vi "find_goal_pose.vi"(6 "Reset":bool, 7 "Parameters":T2={"Stimulus"={"Type"=enum."Off", "Phase"=0.0, "Amplitude"=[], "Injection point"=enum."Total pose", "Closed loop"=FALSE, "Offset"=[], "Tip -> world"=FALSE, "Frequency"=0.0, "Length"=0.0}, "Goal Filter A"={"Speedup max"=0.0, "Speedup thresh"=0.0, "Speedup nonlin"=0.0, "Filters"=[]}, "Mode controls"={"Hold"=FALSE, "Cancellation"=FALSE, "Goal filter"=FALSE, "Trigger"=FALSE}, "Manipulator type"=enum."Current piezo", "Manipulator calibration"={"Tool offsets"=[[0.0, 0.0, 36200.0]], "Handle light calibration"=[], "Base pivots"=[], "Output pivots"=[], "Length center"=0.0, "Workspace height"=[], "Workspace diameter"=[0.0, 0.0, 36200.0], "Stack travel"=400.0, "Saturation pos"=375.0, "Inverse filters"=[], "Strut length"=0.0}, "Network"={"Remote Host"="", "Send Status"=FALSE, "Send Port"=0, "Recv Commands"=FALSE, "Recv Port"=0}, "Goal Filter B"={"Speedup max"=0.0, "Speedup thresh"=0.0, "Speedup nonlin"=0.0, "Filters"=[]}, "Cancellation"={"KP"={"XY"=0.0, "Rxy"=0.0, "Z"=0.0, "Rz"=0.0}, "KI"=0.0, "KD"={"XY"=0.0, "Rxy"=0.0, "Z"=0.0, "Rz"=0.0}, "Max vel"=20.0, "Max acc"=0.001, "Int error limit"=3.0, "RCM gain"=0.0, "Bypass"=FALSE, "Degraded gain"=0.0}, "Transition time"=0.0, "Estimation"={"Link"={"Measure noise"=[], "Process noise"=[], "Alt process noise"=[], "Alt turnoff cycles"=20, "Innovation limit"=[], "Residue threshold"=0.0, "Enable"=FALSE}, "Handle"={"Measure noise"=[], "Process noise"=[], "State limits"=[], "Innovation limit"=[], "Prediction Lookahead"=0.0, "Enable"=FALSE}}} {"Transition time" format="%_3f"; "Cancellation"."Degraded gain" min=0 max=1 step=0.1 format="%#_3p"; "Cancellation"."RCM gain" min=0 max=1 step=0.1 format="%#_3p"; "Cancellation"."KD"."Rz" min=-1 max=1 step=0.01 format="%#_3p"; "Cancellation"."KD"."Rxy" min=-1 max=1 step=0.01 format="%#_3p"; "Cancellation"."KD"."Z" min=-1 max=1 step=0.01 format="%#_3p"; "Cancellation"."KD"."XY" min=-1 max=1 step=0.01 format="%#_3p"; "Cancellation"."KI" min=0 max=1 step=0.01 format="%#_3p"; "Cancellation"."KP"."Rz" min=-1 max=1 step=0.01 format="%#_3p"; "Cancellation"."KP"."Rxy" min=-1 max=1 step=0.01 format="%#_3p"; "Cancellation"."KP"."Z" min=-1 max=1 step=0.01 format="%#_3p"; "Cancellation"."KP"."XY" min=-1 max=1 step=0.01 format="%#_3p"; "Cancellation"."Max acc" format="%#_3p"; "Goal Filter B"."Filters"."V limit range" format="%_3p"; "Goal Filter B"."Filters"."V limit" format="%_3p"; "Goal Filter B"."Filters"."Upper Q" format="%_3f"; "Goal Filter B"."Filters"."Upper Fc" format="%_3p"; "Goal Filter B"."Filters"."Lower Q" format="%_3f"; "Goal Filter B"."Filters"."Scale factor" format="%_3f"; "Goal Filter B"."Filters"."Lower Fc" format="%_3p"; "Goal Filter B"."Speedup nonlin" format="%_3p"; "Goal Filter B"."Speedup thresh" format="%_3p"; "Goal Filter B"."Speedup max" format="%_3p"; "Manipulator calibration"."Strut length" format="%#_4p"; "Manipulator calibration"."Saturation pos" format="%#.1f"; "Manipulator calibration"."Stack travel" format="%#.1f"; "Manipulator calibration"."Length center" format="%#_4p"; "Manipulator calibration"."Output pivots" format="%#_6f"; "Manipulator calibration"."Base pivots" format="%#_6f"; "Manipulator calibration"."Handle light calibration" format="%#.1f"; "Goal Filter A"."Filters"."V limit range" format="%_3p"; "Goal Filter A"."Filters"."V limit" format="%_3p"; "Goal Filter A"."Filters"."Upper Q" format="%_3f"; "Goal Filter A"."Filters"."Upper Fc" format="%_3p"; "Goal Filter A"."Filters"."Lower Q" format="%_3f"; "Goal Filter A"."Filters"."Scale factor" format="%_3f"; "Goal Filter A"."Filters"."Lower Fc" format="%_3p"; "Goal Filter A"."Speedup nonlin" format="%_3p"; "Goal Filter A"."Speedup thresh" format="%_3p"; "Goal Filter A"."Speedup max" format="%_3p"; "Stimulus"."Length" min=0.0 max=100.0 step=100.0 format="%#_4p"; "Stimulus"."Frequency" min=0.0 step=100.0 format="%#_4g"; "Stimulus"."Offset" format="%#_3p"; "Stimulus"."Amplitude" format="%#_3p"; "Stimulus"."Phase" min=-180.0 max=360.0 step=100.0 format="%#.2f"}, 10 "Goal position":sgl[][](array[numeric]) format="%#_6p") -> (0 "Saturation":bool[](array[boolean]), 2 "Goal pose":T1 format="%#_5g")   [LabVIEW 2014]
uses:
  testing/Micron params.ctl
  testing/stimulus.ctl
  testing/injection_point.ctl
  goal_loop_parms.ctl
  testing/mode_conrols.ctl
  testing/manipulator_cal.ctl
  asap/labview/testing/probe_calibration.ctl
  host/network_params.ctl
  cancellation/sq_control_params.ctl
  cancellation/decoupled_gain.ctl
  cancellation/estimation_controls.ctl
  <vilib>/Analysis/Matrix/Datatypes/RealMatrix.ctl
  <vilib>/Analysis/baseanly.llb/A x Vector.vi
  <vilib>/Analysis/baseanly.llb/Real A x B.vi
  <vilib>/Analysis/Matrix/Numeric/Conversions/Array To Matrix - RA2.vi
  <vilib>/Analysis/NI_AALBase.lvlib
  <vilib>/Analysis/Matrix/NI_Matrix.lvlib
panel:
  out "KC sat 2":bool[](array[boolean])
  out "Circle sat":bool
  out "KC sat 1":bool[](array[boolean])
  # "True if tip or RCM goal was moved to fit inside the workspace"
  # "Debug:"
  # "Find goal pose given tip and RCM goal points.   This is the output pose that we want the manipulator to move into.\nSee block diagram for details on how 6DOF pose is computed from this 5DOF information (given that the distance from RCM to tip is fixed.)  We also prevent manipulator saturation by compromising the goal to fit inside the design workspace.  This is distinct from the link-length goal substituion done by the position servo loop (which should be in effect for a most a short time if this code is working properly.)"
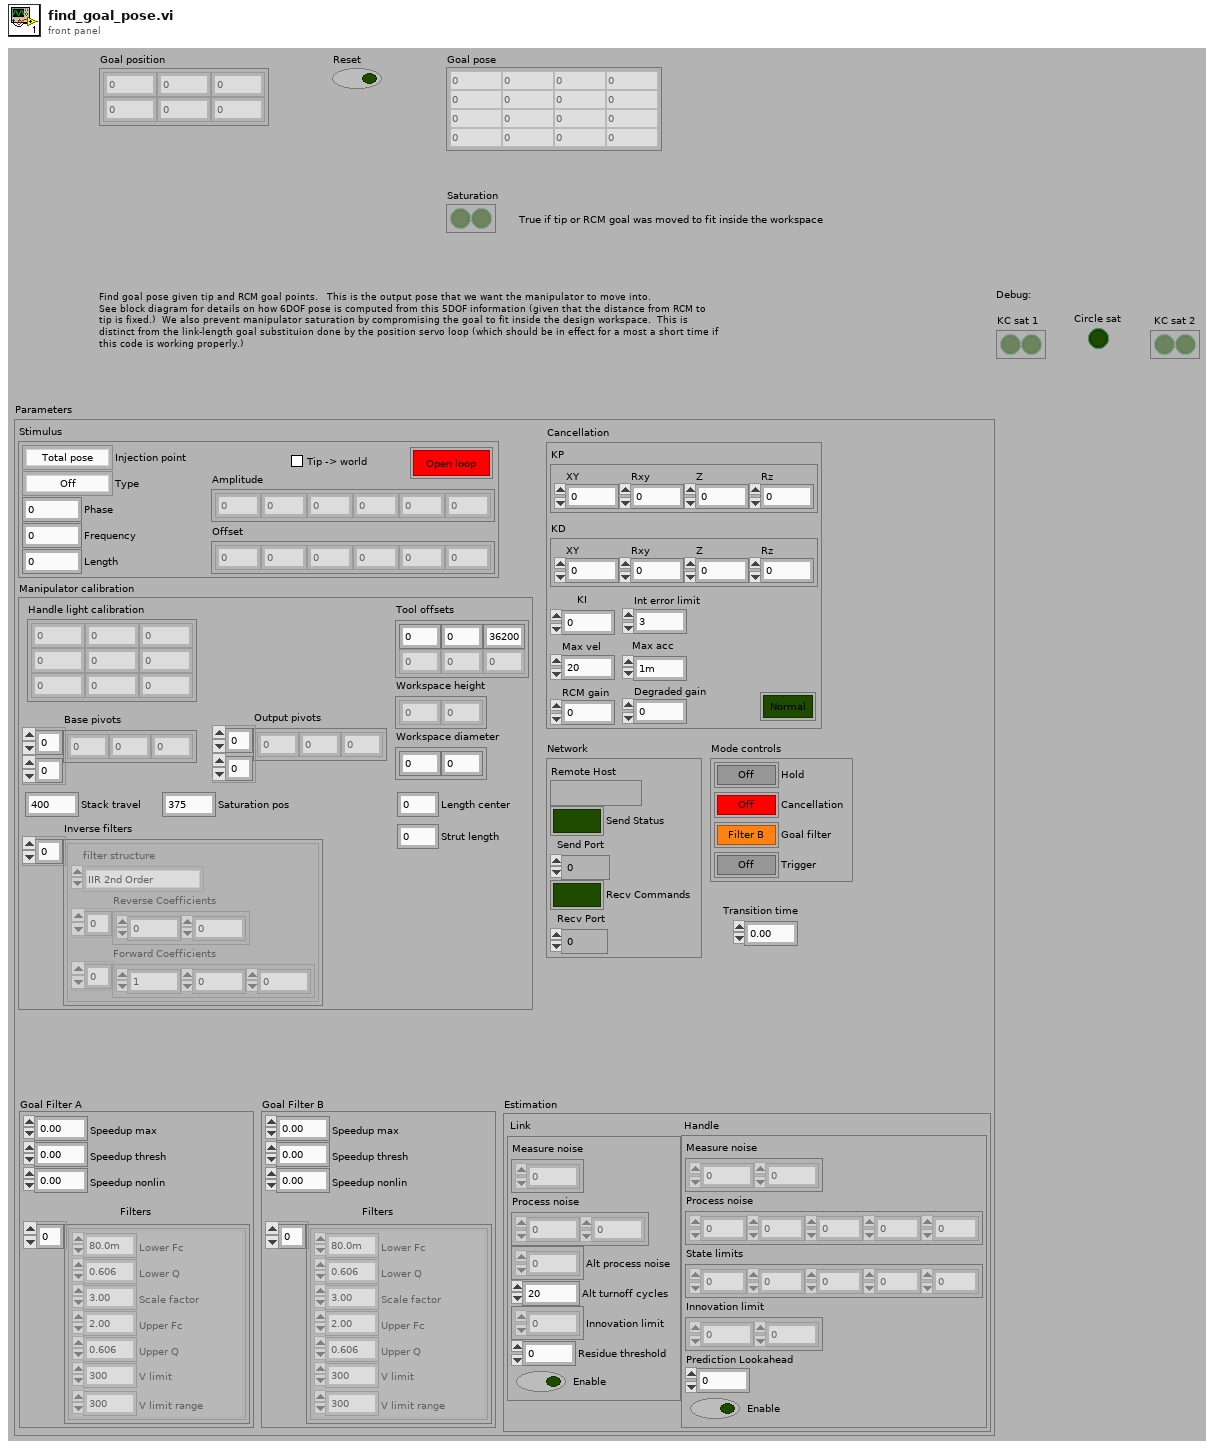
[diagram p1: front panel]
types:
  T1 = typedef "NI_Matrix.lvlib/RealMatrix.ctl" = dbl[][]
  T2 = typedef "Micron params.ctl" = cluster{"Stimulus":T3, "Goal Filter A":T5, "Mode controls":T6, "Manipulator type":enum16{"Current piezo", "Voltage piezo"}, "Manipulator calibration":T7, "Network":T9, "Goal Filter B":T5, "Cancellation":T10, "Transition time":sgl, "Estimation":T12}
  T3 = typedef "stimulus.ctl" = cluster{"Type":enum16{"Off", "Step", "Sine", "Triangle", "Arbitrary"}, "Phase":dbl, "Amplitude":sgl[], "Injection point":T4, "Closed loop":bool, "Offset":sgl[], "Tip -> world":bool, "Frequency":dbl, "Length":dbl}
  T4 = typedef "injection_point.ctl" = enum16{"Total pose", "V limiter", "Goal ", "Link position", "KF link position", "Inverse kin", "Link goal", "Link error", "Controller", "Output", "Drive", "Light"}
  T5 = typedef "goal_loop_parms.ctl" = cluster{"Speedup max":sgl, "Speedup thresh":sgl, "Speedup nonlin":sgl, "Filters":cluster{"Lower Fc":sgl, "Lower Q":sgl, "Scale factor":sgl, "Upper Fc":sgl, "Upper Q":sgl, "V limit":sgl, "V limit range":sgl}[]}
  T6 = typedef "mode_conrols.ctl" = cluster{"Hold":bool, "Cancellation":bool, "Goal filter":bool, "Trigger":bool}
  T7 = typedef "manipulator_cal.ctl" = cluster{"Tool offsets":sgl[][], "Handle light calibration":T8, "Base pivots":sgl[][], "Output pivots":sgl[][], "Length center":sgl, "Workspace height":sgl[], "Workspace diameter":sgl[], "Stack travel":sgl, "Saturation pos":sgl, "Inverse filters":cluster{"filter structure":enum32{"IIR 2nd Order", "IIR 4th Order"}, "Reverse Coefficients":dbl[], "Forward Coefficients":dbl[]}[], "Strut length":sgl}
  T8 = typedef "probe_calibration.ctl" = sgl[][]
  T9 = typedef "network_params.ctl" = cluster{"Remote Host":string, "Send Status":bool, "Send Port":u16, "Recv Commands":bool, "Recv Port":u16}
  T10 = typedef "sq_control_params.ctl" = cluster{"KP":T11, "KI":sgl, "KD":T11, "Max vel":sgl, "Max acc":sgl, "Int error limit":sgl, "RCM gain":sgl, "Bypass":bool, "Degraded gain":sgl}
  T11 = typedef "decoupled_gain.ctl" = cluster{"XY":sgl, "Rxy":sgl, "Z":sgl, "Rz":sgl}
  T12 = typedef "estimation_controls.ctl" = cluster{"Link":cluster{"Measure noise":dbl[], "Process noise":dbl[], "Alt process noise":dbl[], "Alt turnoff cycles":i32, "Innovation limit":dbl[], "Residue threshold":dbl, "Enable":bool}, "Handle":cluster{"Measure noise":dbl[], "Process noise":dbl[], "State limits":dbl[], "Innovation limit":dbl[], "Prediction Lookahead":sgl, "Enable":bool}}
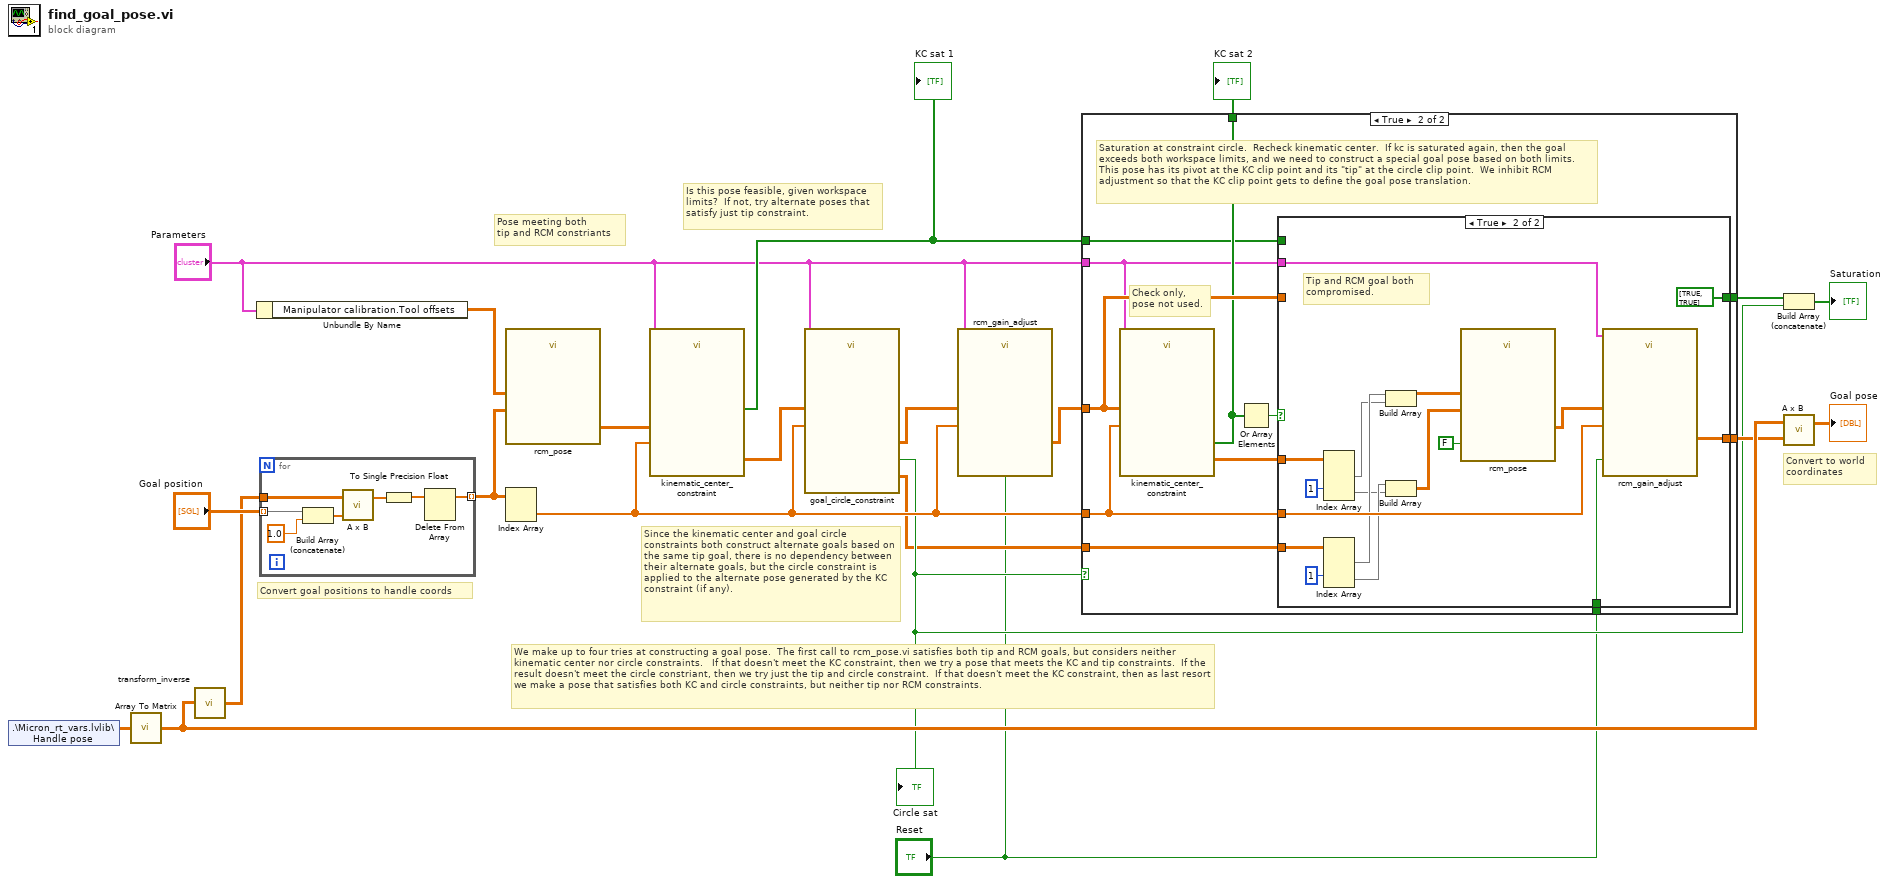
[diagram p0: block diagram]
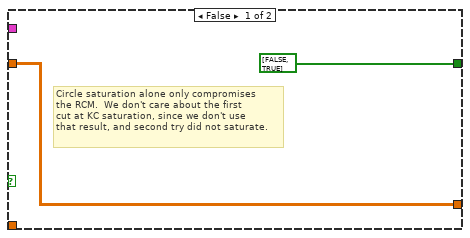
[diagram p3: hidden frame]
diagram:
  # "We make up to four tries at constructing a goal pose.  The first call to rcm_pose.vi satisfies both tip and RCM goals, but considers neither kinematic center nor circle constraints.   If that doesn't meet the KC constraint, then we try a pose that meets the KC and tip constraints.  If the result doesn't meet the circle constriant, then we try just the tip and circle constraint.  If that doesn't meet the KC constraint, then as last resort we make a pose that satisfies both KC and circle constraints, but neither tip nor RCM constraints."
  # "Is this pose feasible, given workspace\nlimits?  If not, try alternate poses that\nsatisfy just tip constraint."
  # "Pose meeting both\ntip and RCM constriants"
  # "Since the kinematic center and goal circle constraints both construct alternate goals based on the same tip goal, there is no dependency between their alternate goals, but the circle constraint is applied to the alternate pose generated by the KC constraint (if any)."
  # "Convert to world\ncoordinates"
  # "Convert goal positions to handle coords"
  n1 = shared-variable ".\\Micron_rt_vars.lvlib\\Handle pose"() -> (w12:sgl[][])  [unwired: 2 out]
  n2 = call-poly <vilib>:"Array To Matrix.vi"("Real 2D Array"=w12) -> ("Real Matrix"=w20:T1)
  n3 = call "transform_inverse.vi"("Transform"=w20) -> ("Inverse transform"=w10:T1)
  n4 = Unbundle By Name("Parameters") -> ("Manipulator calibration.Tool offsets"=w19:sgl[][])
  n5 = for {
    tunnel: [w28] -> w18 mode=indexing
    tunnel: "Goal position" -> [w24] mode=indexing
    tunnel: w10 -> [w23]
    n6 = Build Array (concatenate)(w24, sgl 1.0) -> (w26:sgl[])
    n7 = call-poly <vilib>:"A x B.vi"("Vector"=w26, "A"=w23) -> ("A x Vector"=w22:dbl[])  [unwired: 1 out]
    n8 = To Single Precision Float(number=w22) -> (single precision float=w27:sgl[])
    n9 = Delete From Array(array=w27) -> (array with subset deleted=w28:sgl[])  [unwired: 2 in, 1 out]
  }
  n10 = call "rcm_pose.vi"("Goal positions"=w18, "Nominal positions"=w19) -> ("Goal pose (handle basis)"=w17:T1)  [unwired: 9 in]
  n11 = Index Array(array=w18) -> (element=w7:sgl[])  [unwired: 2 in]
  n12 = call "kinematic_center_constraint.vi"("Goal tip pos"=w7, "Goal pose (handle basis) in"=w17, "Parameters"="Parameters") -> ("Saturation"=w15:bool[], "Goal pose (handle basis) out"=w16:T1)  [unwired: 6 in, 1 out]
  "KC sat 1" <- w15
  n13 = call "goal_circle_constraint.vi"("Goal tip pos"=w7, "Goal pose (handle basis) in"=w16, "Parameters"="Parameters") -> ("Saturation"=w5:bool, "Goal pose (handle basis) out"=w8:T1, "Clip point"=w2:sgl[][])  [unwired: 6 in]
  "Circle sat" <- w5
  n14 = call "rcm_gain_adjust.vi"("Reset"="Reset", "Goal tip pos"=w7, "Goal pose (handle basis) in"=w8, "Parameters"="Parameters") -> ("Goal pose (handle basis) out"=w6:T1)  [unwired: 7 in]
  n15 = case shown="True" w5 {
    tunnel: w6 -> [w30 w38]
    tunnel: [w30 w39] -> w14
    tunnel: w7 -> [_ w34]
    tunnel: "Parameters" -> [_ w33]
    tunnel: w2 -> [_ w41]
    tunnel: w15 -> [w29 w35]
    tunnel: [_ w37] -> w13
    tunnel: [w29 w36] -> w4
    tunnel: "Reset" -> [_ w31]
    frame False {
      # "No circle saturation"
      # "Might have been KC saturation"
    }
    frame True {
      # "Saturation at constraint circle.  Recheck kinematic center.  If kc is saturated again, then the goal exceeds both workspace limits, and we need to construct a special goal pose based on both limits.  This pose has its pivot at the KC clip point and its \"tip\" at the circle clip point.  We inhibit RCM adjustment so that the KC clip point gets to define the goal pose translation."
      # "Check only,\npose not used."
      n16 = call "kinematic_center_constraint.vi"("Goal tip pos"=w34, "Goal pose (handle basis) in"=w38, "Parameters"=w33) -> ("Saturation"=w37:bool[], "Clip point"=w32:sgl[][])  [unwired: 6 in, 1 out]
      n17 = Or Array Elements(Boolean array=w37) -> (logical OR=w40:bool)
      n18 = case shown="True" w40 {
        tunnel: w32 -> [_ w60]
        tunnel: w41 -> [_ w53]
        tunnel: [w43 w58] -> w39
        tunnel: w38 -> [w43 _]
        tunnel: [bool[] [FALSE, TRUE] ("Saturation") bool[] [TRUE, TRUE] ("Saturation")] -> w36
        tunnel: w35 -> [_ _]
        tunnel: w34 -> [_ w56]
        tunnel: w33 -> [_ w57]
        tunnel: w31 -> [_ w44]
        frame False {
          # "Circle saturation alone only compromises\nthe RCM.  We don't care about the first\ncut at KC saturation, since we don't use\nthat result, and second try did not saturate."
        }
        frame True {
          # "Tip and RCM goal both\ncompromised."
          n19 = Index Array(array=w60, index (row) #2=1 ("index (row)")) -> (element #1=w47:sgl[], element #2=w45:sgl[])  [unwired: 3 in]
          n20 = Index Array(array=w53, index (row) #2=1 ("index (row)")) -> (element #1=w48:sgl[], element #2=w46:sgl[])  [unwired: 3 in]
          n21 = Build Array(w48, w47) -> (w52:sgl[][])
          n22 = Build Array(w46, w45) -> (w51:sgl[][])
          n23 = call "rcm_pose.vi"("Adjust RCM"=FALSE, "Goal positions"=w51, "Nominal positions"=w52) -> ("Goal pose (handle basis)"=w49:T1)  [unwired: 8 in]
          n24 = call "rcm_gain_adjust.vi"("Reset"=w44, "Goal tip pos"=w56, "Goal pose (handle basis) in"=w49, "Parameters"=w57) -> ("Goal pose (handle basis) out"=w58:T1)  [unwired: 7 in]
        }
      }
    }
  }
  "KC sat 2" <- w13
  n25 = Build Array (concatenate)(w4, w5) -> (→"Saturation":bool[])
  n26 = call-poly <vilib>:"A x B.vi"("B"=w14, "A"=w20) -> ("A x B"=→"Goal pose":T1)  [unwired: 1 out]
